vi "test Create Default Tag.vi"(8 "error in (no error)":errorcluster, 11 "TestCase in":refnum<class "TagTests.lvclass">) -> (0 "error out":errorcluster, 3 "TestCase out":refnum<class "TagTests.lvclass">)   [LabVIEW 2014, in "TagTests.lvclass"]
uses:
  TagTests.lvclass
  SPLAT/Tag.lvclass
  <vilib>/addons/_JKI Toolkits/VI Tester/TestCase.llb/TestCase.lvclass
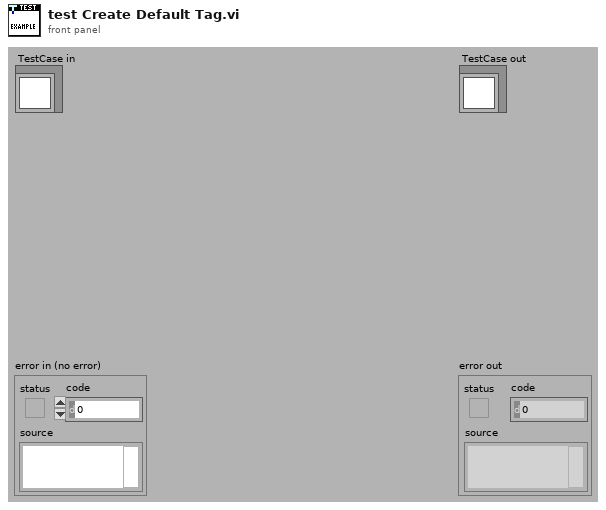
[diagram p1: front panel]
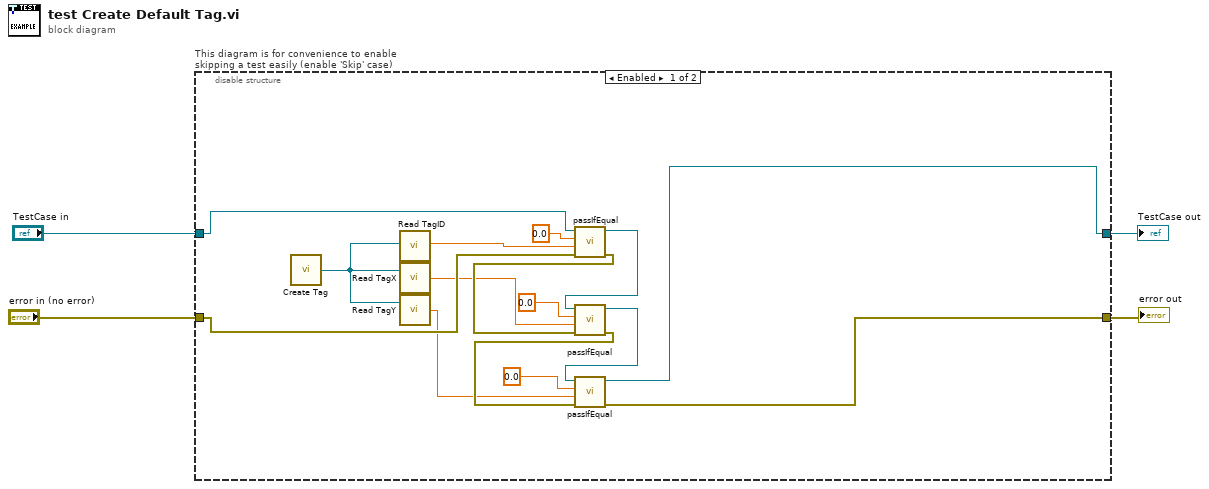
[diagram p0: block diagram]
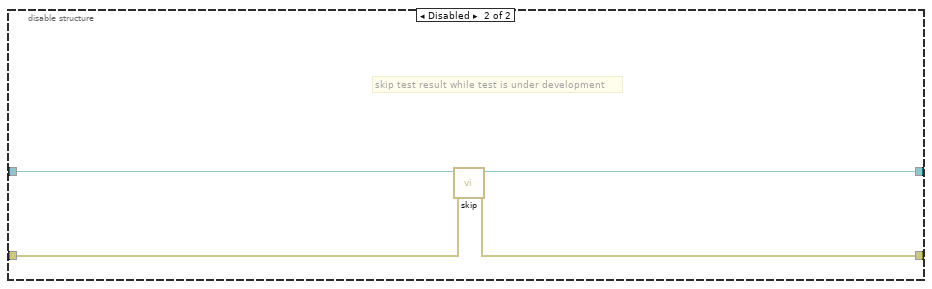
[diagram p2: hidden frame]
diagram:
  n1 = disable-structure "This diagram is for convenience to enable skipping a test easily (enable 'Skip' case)" shown="Enabled" {
    disable-tunnel: "TestCase in" -> [w16 w23]
    disable-tunnel: [w13 w21] -> w1
    disable-tunnel: [w5 w22] -> w3
    disable-tunnel: "error in (no error)" -> [w12 w20]
    frame Enabled {
      n2 = call "Create Tag.vi"() -> ("Tag Out"=w19:refnum<class "Tag.lvclass">)  [unwired: 3 in]
      n3 = call "Read TagID.vi"("Tag in"=w19) -> ("TagID"=w18:dbl)  [unwired: 16 in, 2 out]
      n4 = call-dynamic "Read TagX.vi"("Tag in"=w19) -> ("RealTagX"=w7:dbl)  [unwired: 1 in, 2 out]
      n5 = call-dynamic "Read TagY.vi"("Tag in"=w19) -> ("RealTagY"=w6:dbl)  [unwired: 1 in, 2 out]
      n6 = call-dynamic "passIfEqual.vi"("error in (no error)"=w12, "y"=w18, "x"=0.0, "TestCase in"=w16) -> ("error out"=w11:errorcluster, "TestCase out"=w15:refnum<class "TagTests.lvclass">)  [unwired: 6 in]
      n7 = call-dynamic "passIfEqual.vi"("error in (no error)"=w11, "y"=w7, "x"=0.0, "TestCase in"=w15) -> ("error out"=w10:errorcluster, "TestCase out"=w14:refnum<class "TagTests.lvclass">)  [unwired: 6 in]
      n8 = call-dynamic "passIfEqual.vi"("error in (no error)"=w10, "y"=w6, "x"=0.0, "TestCase in"=w14) -> ("error out"=w5:errorcluster, "TestCase out"=w13:refnum<class "TagTests.lvclass">)  [unwired: 6 in]
    }
    frame Disabled {
      # "skip test result while test is under development"
      n9 = call <vilib>:"skip.vi"("error in (no error)"=w20, "TestCase in"=w23) -> ("error out"=w22:errorcluster, "TestCase out"=w21:refnum<class "TagTests.lvclass">)  [unwired: 8 in]
    }
  }
  "error out" <- w3
  "TestCase out" <- w1
